vi "Fuse.vi"() -> ()   [LabVIEW 2010]
uses:
  PCAN/Labview/ControlCAN/ControlCAN.llb/CAN Channel.ctl
  PCAN/Labview/ControlCAN/ControlCAN.llb/DevType.ctl
  PCAN/Labview/ControlCAN/ControlCAN.llb/VCI_INIT_CONFIG.ctl
  PCAN/Labview/ControlCAN/ControlCAN.llb/InitFlag.ctl
  PCAN/Labview/ControlCAN/ControlCAN.llb/Fliter.ctl
  PCAN/Labview/ControlCAN/ControlCAN.llb/Mode.ctl
  PCAN/Labview/ControlCAN/ControlCAN.lvlib
panel:
  in  "Address":string="192.168.1.2"
  out "TX status":bool
  in  "stop Listen":bool
  in  "status":bool
  in  "Port":u16=8030
  out "conn ID":refnum<k5>
  in  "status 2":bool
  out "Config_CANAT":T7 {"DevType" items=["USB-CAN"=3, "USB-CAN2"=4]; "CanIndex" items=["通道1", "通道2"]; "VCI_INIT_CONFIG"."Fliter" items=["接收所有类型"=3, "只接收标准帧"=4, "只接收扩展帧"=7]; "VCI_INIT_CONFIG"."Mode" items=["正常工作", "自测模式（环回）", "仅侦听模式"]; "VCI_INIT_CONFIG"."InitFlag" items=["使用Flash参数", "使用界面设置参数"]}
  in  "Channel 2":T2 caption="Channel" items=["Channel 1", "Channel 2"]
  in  "CANType":u16(ring) items=["LAWICEL", "PCAN", "CANalystII", "TCP Client", "TCP Server"]
  in  "Get_Log_Time":i32=-1
  in  "Get_Log_Selector":bool
  out "Rcv_Msg":u8
  out "Send_Msg":bool
  in  "ParamFlagStop 2":bool
  out "error out 7":errorcluster
  in  "SysParamFlagStop":bool
  in  "System_Param_Time":i32=-1
  out "System Param Number":u8=9
  in  "System_Selector":bool
  in  "Ch_Selector":bool
  out "Param Nm":u8=9
  in  "ParamFlagStop":bool
  in  "Ch_Param_Time":i32=-1
  out "error out 2":errorcluster
  in  "Clear History":bool
  in  "Ring":u16(ring) items=["None", "Status", "ADC", "Status&ADC", "Temperature"]
  in  "Time":i32=-1
  out "History":string
  in  "Tab Control":T8(tab)
  in  "cleanPl":bool
  out "XY Graph":cluster{"Time":timestamp, "Data":dbl}[](graph)
  in  "Get Temp":bool
  out "Termistor":dbl format="%#.2g"
  in  "Control  Ch 1":bool
  in  "Status":bool
  in  "Trip Status":u16(ring) items=["Not tripped", "Tripped"]
  in  "Status":bool
  in  "Rsense":dbl
  in  "Gain":dbl
  in  "Get_ADC":bool
  out "ADC Units":dbl
  in  "Vin_Vout":bool
  out "Vin [V]":dbl
  out "Vout [V]":dbl
  in  "System Up Time  Set":u32
  in  "Unit Add Set":u32 format="%.0x"
  in  "R Sense [Ohms] Set":u32
  in  "Op Amp Gain Set":u32
  in  "Set System Params":bool
  in  "Retry Delay Set":u32
  in  "Number Of Retry Set":u32
  in  "Ch Received":u8
  in  "Set Channel Params":bool
  in  "Current Threshold [A] Set":u32
  in  "Channel On Delay [ms] Set":u32
  out "System Up Time":u32
  out "Unit Add":u32 format="%.0x"
  out "R Sense [Ohms]":u32
  out "Op Amp Gain":u32
  in  "Get System Params":bool
  out "Retry Delay":u32
  out "Number Of Retry":u32
  out "Ch Received":u8
  in  "Get Params":bool
  out "Current Threshold [A]":u32
  out "Channel On Delay [ms]":u32
  in  "Get Version":bool
  out "Unit PN":string
  out "SW ver":string
  in  "Clear Log":bool
  out "Event Logs":string
  in  "Get Log":bool
  in  "Clear Event Logs":bool
  out "Reset Fail":u32
  in  "Get Channel Protection":bool
  out "Channel Protection":string
  in  "Set Protection":u8(ring)=1 items=["No Protection"=3, "FF_OFF"=2, "ADC_OFF"=1, "All"=0]
  in  "Channel":u8(ring)=1 items=["Ch 1"=1, "Ch 2"=2, "Ch 3"=3, "Ch 4"=4, "Ch 5"=5, "Ch 6"=6, "Ch 7"=7, "Ch 8"=8]
  in  "Set Channel Protection":bool
  in  "TxID":u32 format="%x"
  in  "Data":u8[](array[numeric]) format="%.0x"
  in  "Sent Debug":bool
  out "MsgRX":T9 {"ID" format="%x"; "MSGTYPE" items=["STATUS"=128, "EXTENDED"=2, "RTR"=1, "DATA MSG"=0]; "aDATA" format="%x"}
  out "MsgTX":T9 {"ID" format="%x"; "MSGTYPE" items=["STATUS"=128, "EXTENDED"=2, "RTR"=1, "DATA MSG"=0]; "aDATA" format="%x"}
  in  "Channel":u8(ring)=1 items=["Ch 1"=1, "Ch 2"=2, "Ch 3"=3, "Ch 4"=4, "Ch 5"=5, "Ch 6"=6, "Ch 7"=7, "Ch 8"=8]
  in  "Get Reset count":bool
  out "Reset Counter":u32
  out "RX Cnt":u32
  out "TX Cnt":u32
  in  "stop m":bool
  out "error out 5":errorcluster
  out "error out 6":errorcluster
  out "erroro5 2":errorcluster
  out "erroro5":errorcluster
  out "error out 4":errorcluster
  out "VISA res_out":refnum<visa-resource-name>
  in  "Seria- Port":refnum<visa-resource-name>="COM5"
  out "error out 3":errorcluster
  out "error02":errorcluster
  out "error out":errorcluster
  out "RX":bool
  out "TX":bool
  in  "Disonnect":bool
  in  "Connect":bool
  out "CommIcon":bool=TRUE
  in  "UIFlagStop":bool
  in  "RXFlagStop":bool
  in  "IntFlagStop":bool
  in  "TXFlagStop":bool
  out "Error":string
  out "Adapter Version":string
  in  "type":i32(ring) items=["extended", "standart"]
  in  "baud":u16(ring)=20 items=["1M"=20, "500K"=28, "250K"=284, "125K"=796, "100K"=17199, "50K"=18223, "20K"=21295, "10K"=26415, "5K"=32639]
  # "[msec]"
  # "ver 0.0.1.b"
  # "Fuse Status"
  # "ADC"
  # "Temperature"
  # "Vin/Vout"
  # "Version"
  # "Channel Parameter"
  # "System Parameters"
  # "Channel Parameter"
  # "System Parameters"
  # "Custom Message"
  # "FF Reset Counter"
  # "Channel Protection"
  # "PowerRider CANBus interface"
  # "REDLER TECHNOLOGIES LTD"
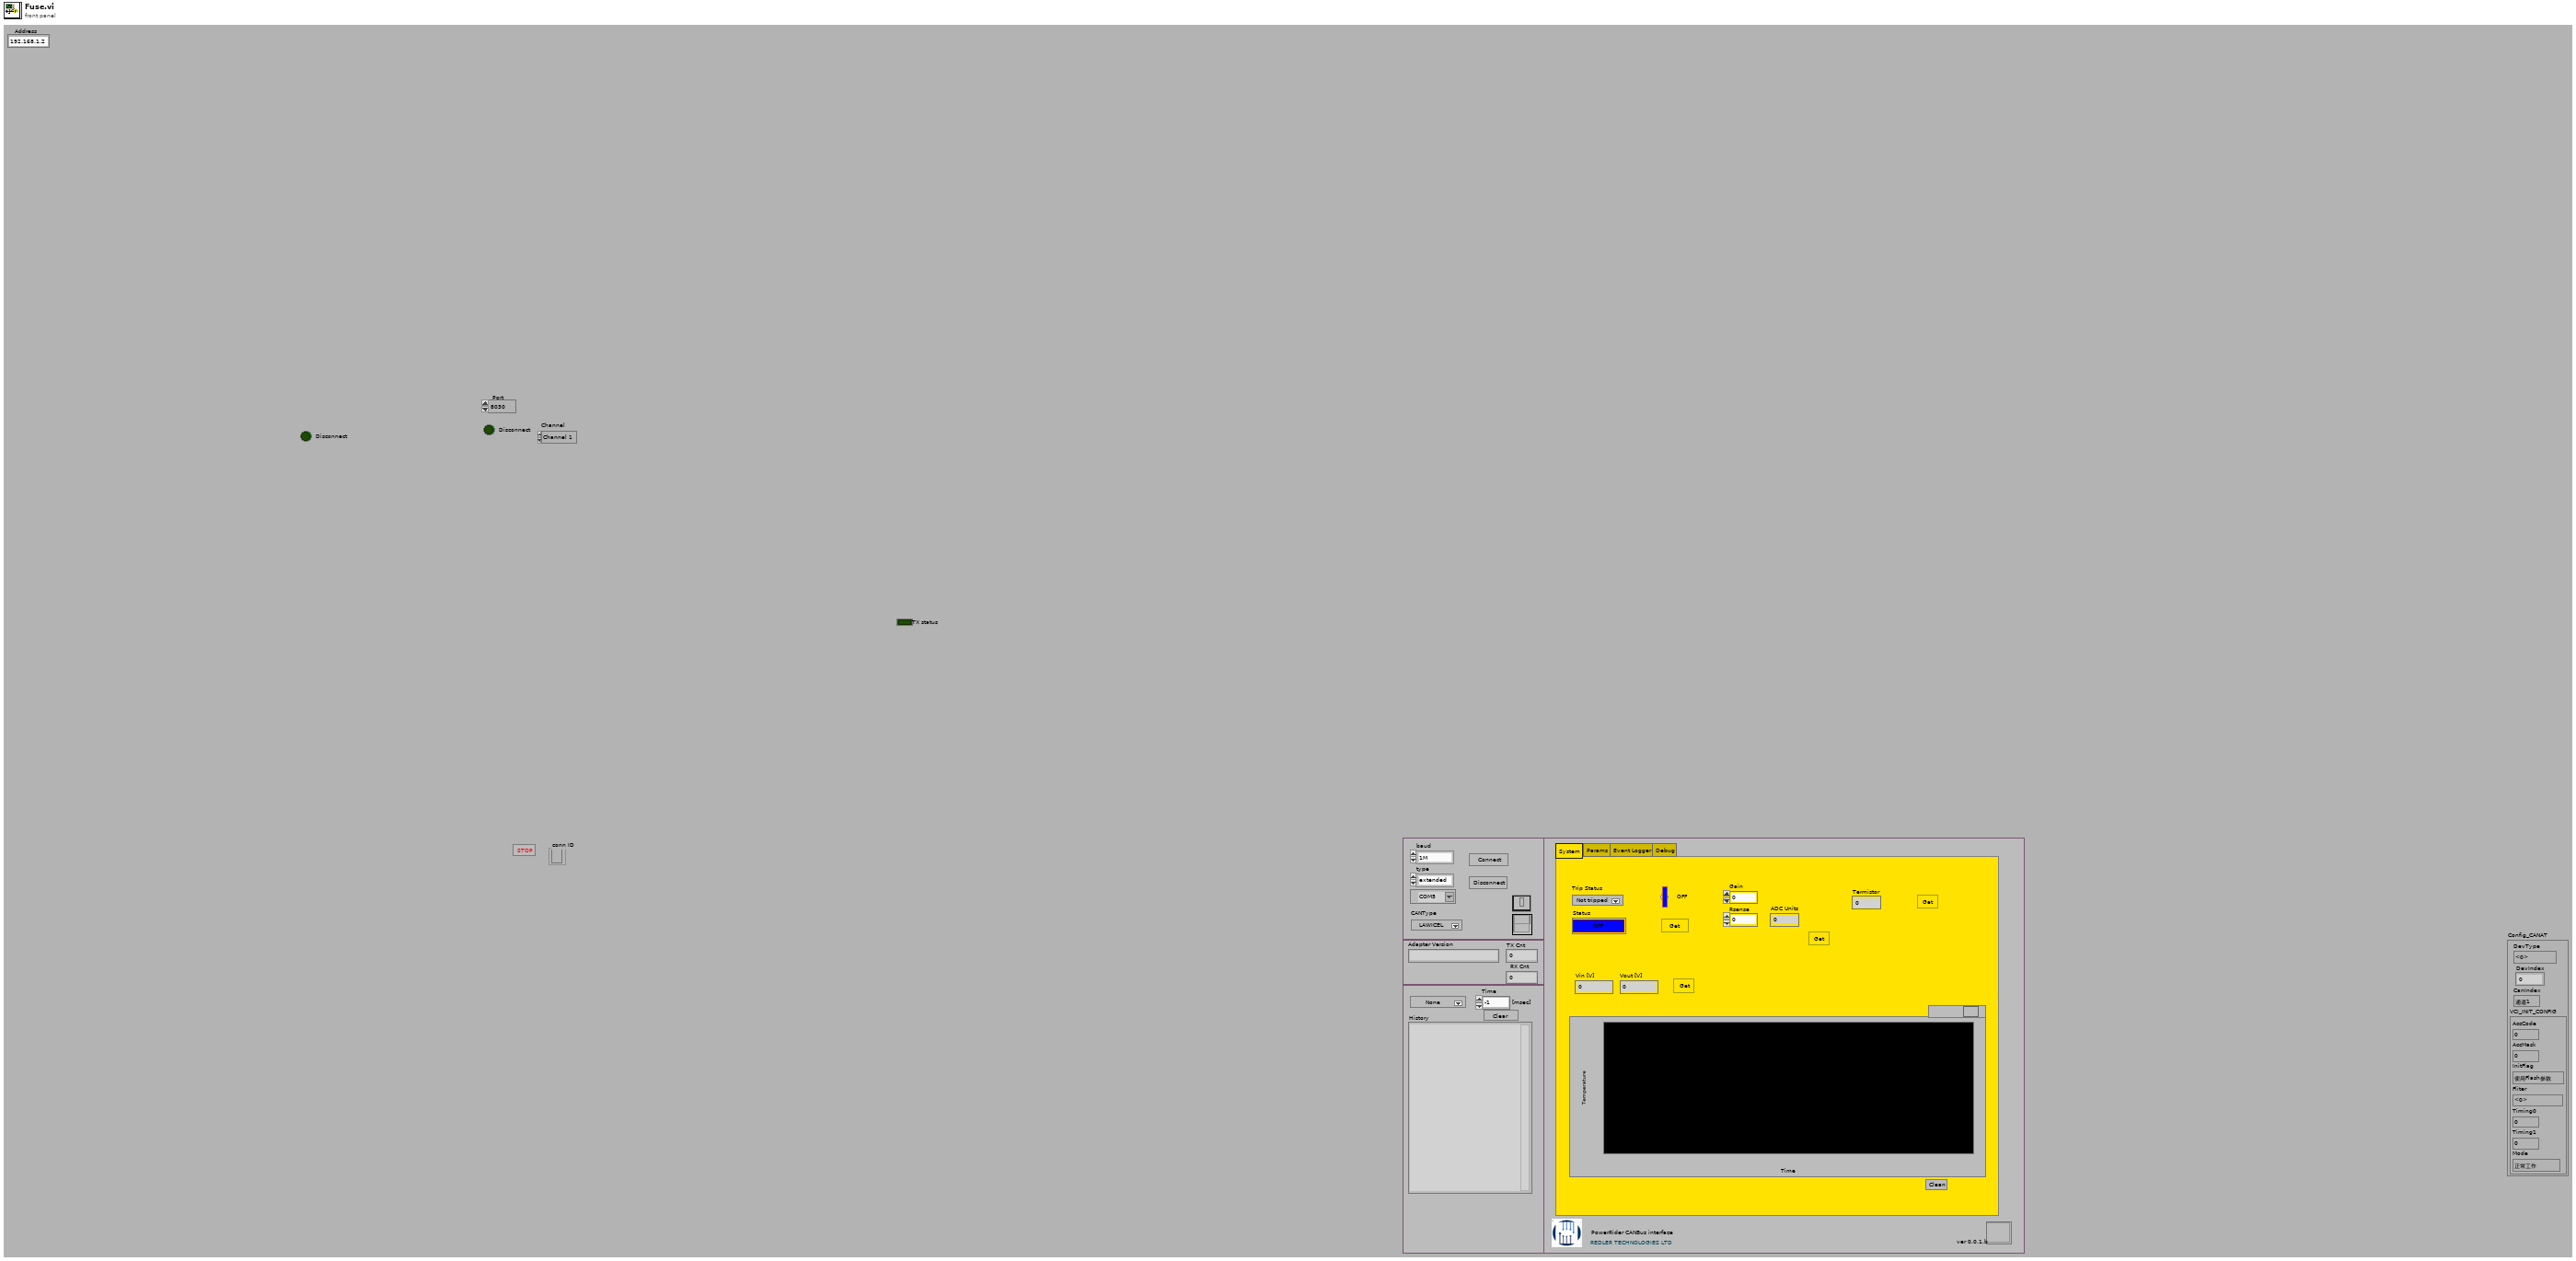
[diagram p1: front panel]
types:
  T1 = typedef "ControlCAN.lvlib/DevType.ctl" = u32
  T2 = typedef "ControlCAN.lvlib/CAN Channel.ctl" = u32
  T3 = typedef "ControlCAN.lvlib/VCI_INIT_CONFIG.ctl" = cluster{"AccCode":u32, "AccMask":u32, "InitFlag":T4, "Fliter":T5, "Timing0":u8, "Timing1":u8, "Mode":T6}
  T4 = typedef "ControlCAN.lvlib/InitFlag.ctl" = u32
  T5 = typedef "ControlCAN.lvlib/Fliter.ctl" = u8
  T6 = typedef "ControlCAN.lvlib/Mode.ctl" = u8
  T7 = cluster{"DevType":T1, "DevIndex":u32, "CanIndex":T2, "VCI_INIT_CONFIG":T3}
  T8 = enum32{"System", "Params", "Event Logger", "Debug"}
  T9 = cluster{"ID":u32, "MSGTYPE":u8, "LEN":u8, "aDATA":u8[]}
  T10 = typedef "PCAN_ERROR.ctl" = i32
  T11 = cluster{"Is Warning":bool, "Is Error":bool, "Message":string}
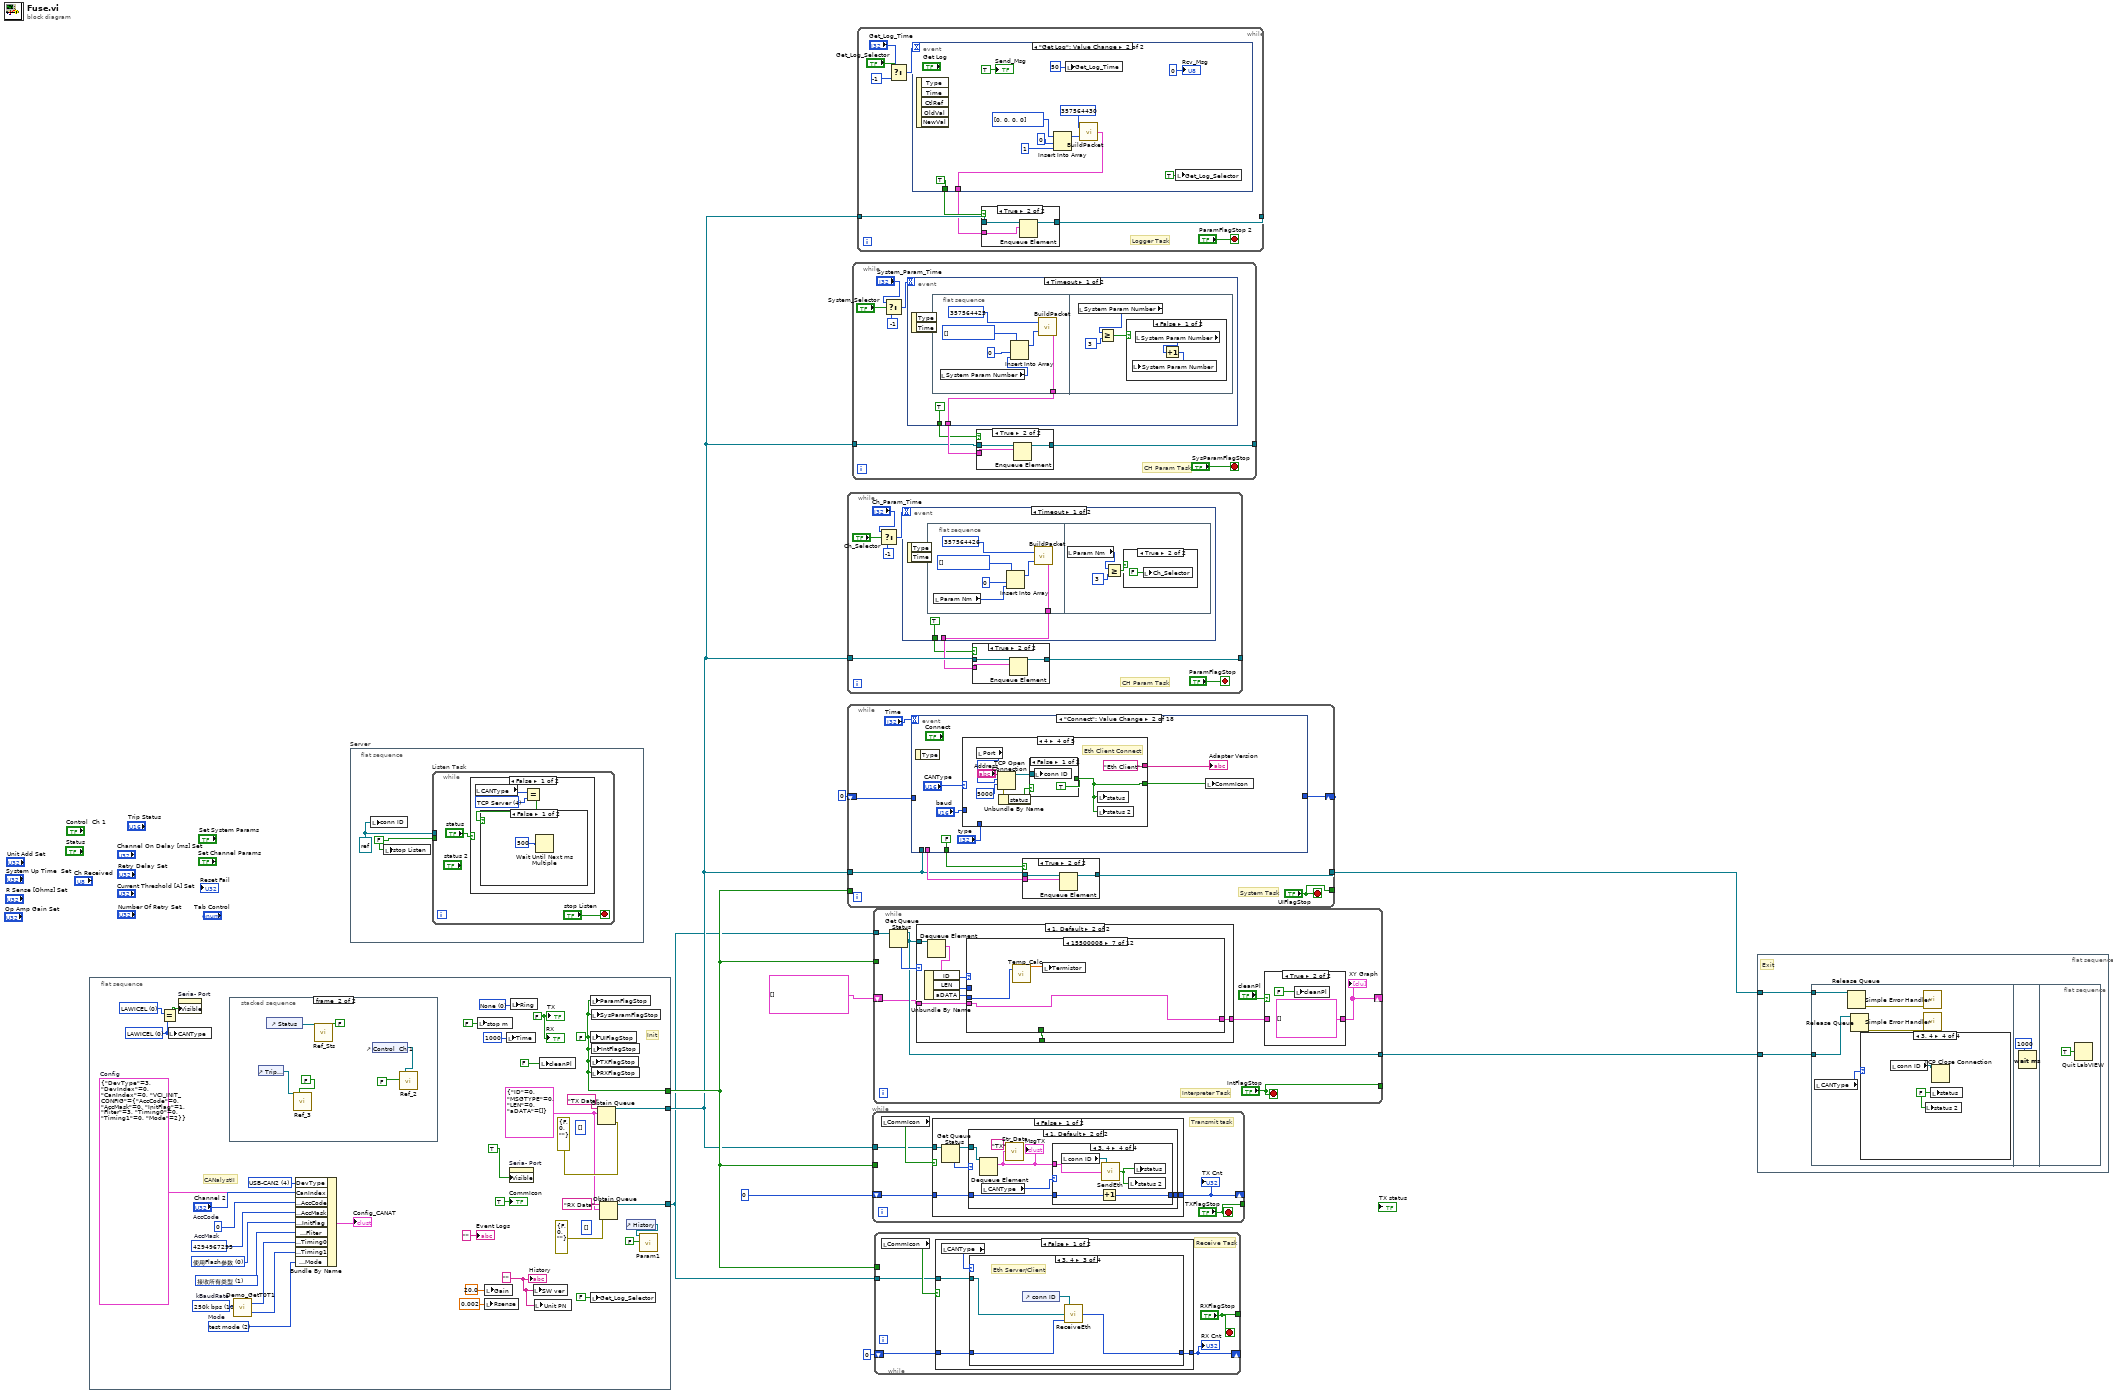
[diagram p0: block diagram]
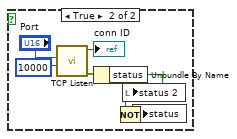
[diagram p2: hidden frame]
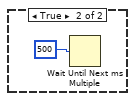
[diagram p3: hidden frame]
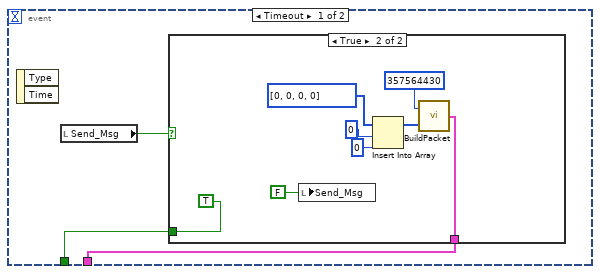
[diagram p4: hidden frame]
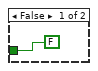
[diagram p5: hidden frame]
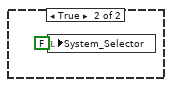
[diagram p7: hidden frame]
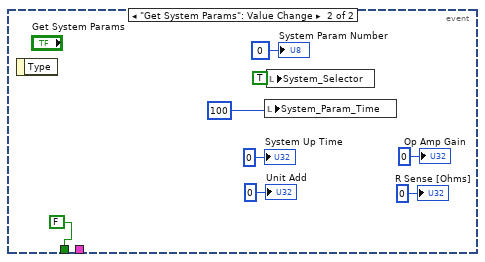
[diagram p8: hidden frame]
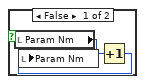
[diagram p10: hidden frame]
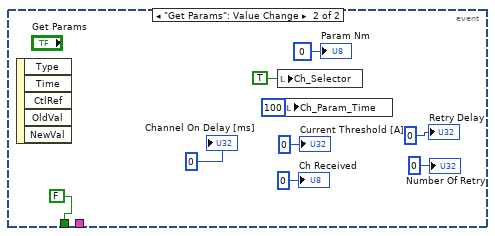
[diagram p11: hidden frame]
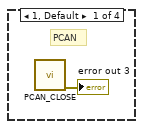
[diagram p13: hidden frame]
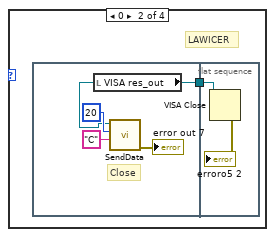
[diagram p14: hidden frame]
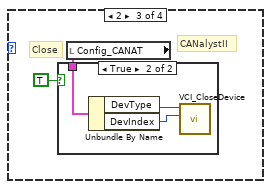
[diagram p15: hidden frame]
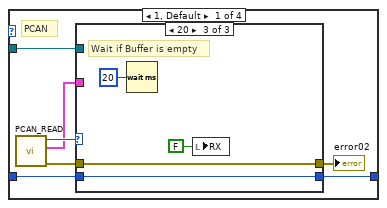
[diagram p17: hidden frame]
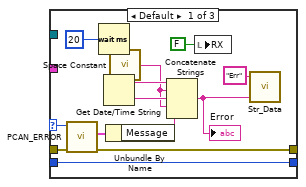
[diagram p18: hidden frame]
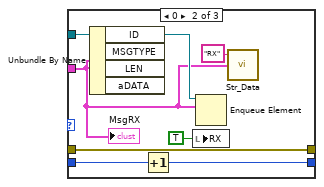
[diagram p19: hidden frame]
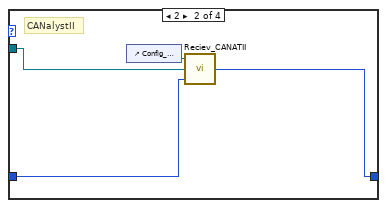
[diagram p20: hidden frame]
diagram:
  n1 = flat-sequence {
    tunnel: [w28] -> w9
    tunnel: [w42] -> w3
    tunnel: [w38] -> w1
    frame #0 {
      w11 = u16 0 items=["LAWICEL", "PCAN", "CANanlII"] ("CANType")
      w17 = u32 4294967295  # AccMask
      w18 = T4 0 items=["使用Flash参数", "使用界面设置参数"] ("InitFlag")
      w23 = T6 2 items=["normal operation", "Listen-only mode", "test mode"]  # Mode
      w19 = T5 1 items=["接收所有类型"=1, "只接收标准帧"=2, "只接收扩展帧"=3] ("Fliter")
      w20 = u8 10 items=["5k bps"=1, "10k bps"=2, "20k bps"=3, "40k bps"=4, "50k bps"=5, "80k bps"=6, "100k bps"=7, "125k bps"=8, "200k bps"=9, "250k bps"=10, "400k bps"=11, "500k bps"=12, "666k bps"=13, "800k bps"=14, "1000k bps"=15, "33.33k bps"=16, "66.66k bps"=17, "83.33k bps"=18]  # kBaudRate
      w16 = u32 0  # AccCode
      w14 = T1 4 items=["USB-CAN"=3, "USB-CAN2"=4] ("DevType")
      w13 = T7 {"DevType"=3, "DevIndex"=0, "CanIndex"=0, "VCI_INIT_CONFIG"={"AccCode"=0, "AccMask"=0, "InitFlag"=1, "Fliter"=3, "Timing0"=0, "Timing1"=0, "Mode"=2}}  # Config
      w12 = u16 0 items=["LAWICEL", "PCAN", "CANanlII"] ("CANType")
      w32 = u16 0 items=["None", "Status", "ADC", "Status&ADC"] ("Ring")
      w31 = "" ("str out")
      w39 = T9 {"ID"=0, "MSGTYPE"=0, "LEN"=0, "aDATA"=[]} ("Msg")
      w40 = FALSE ("TX")
      (unwired) u8[] []
      (unwired) u8[] []
      w28 = FALSE ("UIFlagStop")
      # "CANalystII"
      # "Init"
      n2 = Equal?(x=w11, y=w12) -> (x = y?=w10:bool)
      n3 = local write "CANType"(w12) -> ()
      n4 = property on="Seria- Port" class="VISAName"("Visible"=w10) -> ()  [unwired: 2 in, 2 out]
      n5 = stacked-sequence {
        frame #0 {
          n6 = local write "Control  Ch 1"(FALSE ("Control  Ch 1")) -> ()
          n7 = local write "Status"(FALSE ("Status")) -> ()
        }
        frame #1 {
          n8 = control-ref of="Trip Status"() -> (w50:refnum<vi>)
          n9 = control-ref of="Status"() -> (w52:refnum<vi>)
          n10 = call "Ref_3.vi"("Trip  Ch 1"=w50, "Init_F"=FALSE) -> ()  [unwired: 16 in, 10 out]
          n11 = call "Ref_Sts.vi"("Status Ch 1"=w52, "Init_F"=FALSE) -> ()  [unwired: 16 in, 10 out]
          n12 = control-ref of="Control  Ch 1"() -> (w54:refnum<vi>)
          n13 = call "Ref_2.vi"("Init_F"=FALSE, "Control  Ch 1"=w54) -> ()  [unwired: 15 in, 11 out]
        }
      }
      n14 = call "Demo_GetT0T1.vi"("kBaudRate"=w20) -> ("Timing0"=w21:u8, "Timing1"=w22:u8)
      n15 = Bundle By Name(cluster=w13, "DevType"=w14, "CanIndex"="Channel 2", "VCI_INIT_CONFIG.AccCode"=w16, "VCI_INIT_CONFIG.AccMask"=w17, "VCI_INIT_CONFIG.InitFlag"=w18, "VCI_INIT_CONFIG.Fliter"=w19, "VCI_INIT_CONFIG.Timing0"=w21, "VCI_INIT_CONFIG.Timing1"=w22, "VCI_INIT_CONFIG.Mode"=w23) -> (→"Config_CANAT":T7)
      n16 = local write "stop m"(FALSE ("stop m")) -> ()
      n17 = local write "Rsense"(0.002 ("Rsense")) -> ()
      n18 = local write "Gain"(20.0 ("Gain")) -> ()
      n19 = local write "Time"(1000 ("Time")) -> ()
      n20 = property on="Seria- Port" class="VISAName"("Visible"=TRUE ("CAN Type")) -> ()  [unwired: 2 in, 2 out]
      n21 = local write "Ring"(w32) -> ()
      n22 = local write "SW ver"(w31) -> ()
      n23 = local write "Unit PN"(w31) -> ()
      n24 = local write "cleanPl"(FALSE ("clean  Ch 2")) -> ()
      n25 = local write "ParamFlagStop"(w28) -> ()
      n26 = local write "UIFlagStop"(w28) -> ()
      n27 = local write "TXFlagStop"(w28) -> ()
      n28 = local write "Get_Log_Selector"(FALSE ("Get_Log_Selector")) -> ()
      n29 = local write "SysParamFlagStop"(w28) -> ()
      n30 = local write "RXFlagStop"(w28) -> ()
      n31 = local write "IntFlagStop"(w28) -> ()
      n32 = Obtain Queue(name (unnamed)="TX Data", element data type=w39, error in (no error)=errorcluster {"status"=FALSE, "code"=0, "source"=""}) -> (queue out=w42:refnum<queue>)  [unwired: 2 in, 2 out]
      n33 = Obtain Queue(name (unnamed)="RX Data", element data type=w39, error in (no error)=errorcluster {"status"=FALSE, "code"=0, "source"=""}) -> (queue out=w38:refnum<queue>)  [unwired: 2 in, 2 out]
      n34 = control-ref of="History"() -> (w34:refnum<vi>)
      n35 = call "Param1.vi"("str"=w34, "Init_F"=FALSE) -> ()  [unwired: 16 in, 2 out]
      "CommIcon" <- TRUE ("CommIcon")
      "RX" <- w40
      "TX" <- w40
      "History" <- w31
      "Event Logs" <- "" ("Event Logs")
    }
  }
  n36 = flat-sequence "Server" {
    frame #0 {
      w56 = refnum<k5> refnum ("connection ID")
      w55 = FALSE ("status")
      n37 = local write "conn ID"(w56) -> ()
      n38 = local write "stop Listen"(w55) -> ()
      n39 = while "Listen Task" {
        tunnel: w55 -> [_]
        tunnel: w56 -> [_]
        stop <- "stop Listen" stop-if-true
        n40 = case shown="False" "status" {
          frame False {
            w60 = u16 4 items=["LAWICEL", "PCAN", "CANalystII", "TCP Client", "TCP Server"] ("CANType 2")
            n41 = local read "CANType"() -> (w61:u16)
            n42 = Equal?(x=w61, y=w60) -> (x = y?=w59:bool)
            n43 = case shown="False" w59 {
              frame False {
                n44 = Wait Until Next ms Multiple(millisecond multiple=u32 500) -> ()  [unwired: 1 out]
              }
              frame True {
                n45 = call <vilib>:"TCP Listen.vi"("timeout ms (wait forever: -1)"=10000, "port"="Port") -> ("error out"=w66:errorcluster, "connection ID"=→"conn ID":refnum<k5>)  [unwired: 6 in, 2 out]
                n46 = Unbundle By Name(w66) -> ("status"=w63:bool)
                n47 = Not(x=w63) -> (.not. x?=w64:bool)
                n48 = local write "status 2"(w63) -> ()
                n49 = local write "status"(w64) -> ()
              }
            }
          }
          frame True {
            n50 = Wait Until Next ms Multiple(millisecond multiple=u32 500) -> ()  [unwired: 1 out]
          }
        }
      }
    }
  }
  n51 = while {
    tunnel: w3 -> [w77]
    tunnel: [w76] -> _
    stop <- "ParamFlagStop" stop-if-true
    # "CH Param Task"
    n52 = Select(t="Ch_Param_Time", s="Ch_Selector", f=-1) -> (s? t:f=w73:i32)
    n53 = event shown="[0] Timeout" {
      selector: _ -> [_ _]
      dyn-events: _ -> [_ _]
      timeout: w73 -> [_ _]
      tunnel: [w80 _] -> w72
      tunnel: [TRUE FALSE] -> w70
      event Timeout {
        n54 = event-data() -> ()  [unwired: 1 in, 2 out]
        n55 = flat-sequence {
          tunnel: [w86] -> w80
          frame #0 {
            n56 = local read "Param Nm"() -> (w81:u8)
            n57 = Insert Into Array(array=u8[] [] ("Data 2"), index=0, new element=w81) -> (w82:u8[])
            n58 = call "BuildPacket.vi"("Data"=w82, "TxID"=u32 357564426 ("Param ID")) -> ("MsgTX 2"=w86:T9)
          }
          frame #1 {
            n59 = local read "Param Nm"() -> (w89:u8)
            n60 = Greater Or Equal?(x=w89, y=u8 3) -> (x >= y?=w88:bool)
            n61 = case shown="True" w88 {
              frame False {
                n62 = local read "Param Nm"() -> (w91:u8)
                n63 = Increment(x=w91) -> (x+1=w90:u8)
                n64 = local write "Param Nm"(w90) -> ()
              }
              frame True {
                n65 = local write "Ch_Selector"(FALSE ("Timer Select")) -> ()
              }
            }
          }
        }
      }
      event "Get Params": Value Change {
        n66 = event-data() -> ()  [unwired: 1 in, 5 out]
        n67 = local write "Ch_Selector"(TRUE ("Timer Select")) -> ()
        n68 = local write "Ch_Param_Time"(100 ("Time Param")) -> ()
        "Param Nm" <- u32 0 ("Param ID")
        "Current Threshold [A]" <- u32 0 ("Current Threshold [A]")
        "Ch Received" <- u8 0 ("Ch Received")
        "Channel On Delay [ms]" <- u32 0 ("Channel On Delay [ms]")
        "Number Of Retry" <- u32 0 ("Ch Received")
        "Retry Delay" <- u32 0 ("Current Threshold [A]")
      }
    }
    n69 = case shown="True" w70 {
      tunnel: w77 -> [w102 w105]
      tunnel: [w102 w104] -> w76
      tunnel: w72 -> [_ w103]
      frame False {
      }
      frame True {
        n70 = Enqueue Element(queue=w105, element=w103) -> (queue out=w104:refnum<queue>)  [unwired: 1 in, 3 out]
      }
    }
  }
  n71 = while {
    tunnel: w9 -> [_]
    tunnel: ["UIFlagStop"] -> _
    tunnel: w3 -> [w107]
    tunnel: [w106] -> w8
    shift-right: [w108] -> _
    shift-left: u32 0 -> [w109]
    stop <- "UIFlagStop" stop-if-true
    # "System Task"
    n72 = event shown="[1] \"Connect\": Value Change" {
      selector: _ -> [_ _ _ _ _ _ _ _ _ _ _ _ _ _ _ _ _ _]
      dyn-events: _ -> [_ _ _ _ _ _ _ _ _ _ _ _ _ _ _ _ _ _]
      timeout: "Time" -> [_ _ _ _ _ _ _ _ _ _ _ _ _ _ _ _ _ _]
      tunnel: [w121 _ _ w192 w197 _ w205 w211 w218 w222 w228 w245 w255 w259 _ _ _ w287] -> w112
      tunnel: [w122 FALSE FALSE TRUE TRUE FALSE TRUE TRUE TRUE TRUE TRUE TRUE TRUE TRUE FALSE FALSE _ TRUE] -> w111
      tunnel: w109 -> [w119 _ _ _ _ w202 _ _ _ _ _ _ _ _ _ _ _ _]
      tunnel: [w118 _ _ _ _ w202 _ _ _ _ _ _ _ _ _ _ _ _] -> w108
      tunnel: w107 -> [_ _ _ _ _ _ _ _ _ _ _ _ _ _ _ _ _ _]
      event Timeout {
        n73 = event-data() -> ()  [unwired: 1 in, 1 out]
        n74 = case shown="3" "Ring" {
          tunnel: [FALSE TRUE TRUE TRUE] -> w122
          tunnel: [T9 {"ID"=0, "MSGTYPE"=0, "LEN"=0, "aDATA"=[]} ("Msg") w127 w132 w138] -> w121
          tunnel: w119 -> [_ _ _ w140]
          tunnel: [u32 0 u32 0 u32 0 w136] -> w118
          frame 0, Default {
          }
          frame 1 {
            w129 = u32 357564416  # ID
            # "Status"
            n75 = call "BuildPacket.vi"("Data"=u8[] [] ("Data 2"), "TxID"=w129) -> ("MsgTX 2"=w127:T9)
          }
          frame 2 {
            w133 = u32 357564419  # ID
            # "ADC"
            n76 = call "BuildPacket.vi"("Data"=u8[] [] ("Data 2"), "TxID"=w133) -> ("MsgTX 2"=w132:T9)
          }
          frame 3 {
            n77 = case shown="1" w140 {
              selector: w140 -> [w143 _]
              tunnel: [w144 w146] -> w137
              tunnel: [w142 u32 0] -> w136
              frame 0, Default {
                w144 = u32 357826560  # ID
                # "Status"
                n78 = Increment(x=w143) -> (x+1=w142:u32)
              }
              frame 1 {
                w146 = u32 357564419  # ID
                # "ADC"
              }
            }
            n79 = call "BuildPacket.vi"("Data"=u8[] [] ("Data 2"), "TxID"=w137) -> ("MsgTX 2"=w138:T9)
          }
        }
      }
      event "Connect": Value Change {
        n80 = event-data() -> ()  [unwired: 1 in, 1 out]
        n81 = case shown="4" "CANType" {
          tunnel: [w155 w162 w168 w171 w182] -> w151
          tunnel: [w157 "CANalystII" ("read ver") "" ("read ver") "Eth Client" ("read ver") w183] -> w150
          tunnel: "baud" -> [w154 w161 _ _ w181]
          tunnel: "type" -> [w153 w160 _ _ _]
          frame 1, Default {
            # "PCAN"
            n82 = call "Init_PCAN.vi"("type"=w153, "baud"=w154) -> ("Boolean"=w156:bool, "Version"=w157:string)
            n83 = Not(x=w156) -> (.not. x?=w155:bool)
          }
          frame 2 {
            # "CANalystII"
            n84 = flat-sequence {
              tunnel: w161 -> [w165]
              tunnel: w160 -> [_]
              tunnel: [w164] -> w158
              tunnel: [w167] -> w159
              tunnel: w158 -> [w166]
              frame #0 {
                n85 = control-ref of="Config_CANAT"() -> (w164:refnum<vi>)
                n86 = call "ChangeCANBaud.vi"("baud in"=w165, "reference"=w164) -> ()
              }
              frame #1 {
                n87 = call "InitCAN_ATII.vi"("Config"=w166) -> ("Sts"=w167:bool)
              }
            }
            n88 = Not(x=w159) -> (.not. x?=w162:bool)
          }
          frame 3 {
            # "Eth Server Connect"
            n89 = local read "CommIcon"() -> (w168:bool)
          }
          frame 4 {
            # "Eth Client Connect"
            n90 = local read "Port"() -> (w175:u16)
            n91 = TCP Open Connection(address="Address", remote port or service name=w175, timeout ms (60000)=5000) -> (connection ID=w177:refnum<k5>, error out=w173:errorcluster)  [unwired: 1 in, 1 out]
            n92 = Unbundle By Name(w173) -> ("status"=w176:bool)
            n93 = case shown="False" w176 {
              tunnel: w177 -> [w179 _]
              tunnel: [TRUE FALSE] -> w171
              frame False {
                n94 = local write "conn ID"(w179) -> ()
              }
              frame True {
              }
            }
            n95 = local write "status"(w171) -> ()
            n96 = local write "status 2"(w171) -> ()
          }
          frame 0 {
            # "LAWICER"
            n97 = call "Init_Lawicel.vi"("baud"=w181, "Seria- Port"="Seria- Port") -> ("error out 4"=→"error out 4":errorcluster, "Status"=w184:bool, "read ver"=w183:string, "VISA res_out"=→"VISA res_out":refnum<visa-resource-name>)  [unwired: 1 in]
            n98 = Not(x=w184) -> (.not. x?=w182:bool)
          }
        }
        "Adapter Version" <- w150
        n99 = local write "CommIcon"(w151) -> ()
      }
      event "stop m": Value Change {
        w188 = TRUE ("UIFlagStop")
        n100 = event-data() -> ()  [unwired: 1 in, 1 out]
        n101 = local write "UIFlagStop"(w188) -> ()
        n102 = local write "TXFlagStop"(w188) -> ()
        n103 = local write "RXFlagStop"(w188) -> ()
        n104 = local write "IntFlagStop"(w188) -> ()
        n105 = local write "SysParamFlagStop"(w188) -> ()
        n106 = local write "ParamFlagStop"(w188) -> ()
      }
      event "Sent Debug": Value Change {
        n107 = event-data() -> ()  [unwired: 1 in, 1 out]
        n108 = call "BuildPacket.vi"("Data"="Data", "TxID"="TxID") -> ("MsgTX 2"=w192:T9)
      }
      event "Get Version": Value Change {
        w194 = "" ("SW ver")
        w195 = u32 357564423  # ID
        # "0x15500007"
        n109 = event-data() -> ()  [unwired: 1 in, 1 out]
        n110 = call "BuildPacket.vi"("Data"=u8[] [] ("Data 2"), "TxID"=w195) -> ("MsgTX 2"=w197:T9)
        "SW ver" <- w194
        "Unit PN" <- w194
      }
      event "CANType": Value Change {
        w200 = u16 0 items=["LAWICEL", "PCAN", "CANanlII"] ("CANType")
        n111 = event-data() -> ()  [unwired: 1 in, 1 out]
        n112 = local read "CANType"() -> (w201:u16)
        n113 = Equal?(x=w200, y=w201) -> (x = y?=w199:bool)
        n114 = property on="Seria- Port" class="VISAName"("Visible"=w199) -> ()  [unwired: 2 in, 2 out]
      }
      event "Get Temp": Value Change {
        w206 = u32 357564424  # ID
        # "0x15500008"
        n115 = event-data() -> ()  [unwired: 1 in, 1 out]
        n116 = call "BuildPacket.vi"("Data"=u8[] [] ("Data 2"), "TxID"=w206) -> ("MsgTX 2"=w205:T9)
        "Termistor" <- 0.0 ("CPU Temp")
      }
      event "Status": Value Change {
        w209 = u32 357564416  # ID
        # "Status"
        # "0x1550000"
        n117 = event-data() -> ()  [unwired: 1 in, 1 out]
        n118 = call "BuildPacket.vi"("Data"=u8[] [] ("Data 2"), "TxID"=w209) -> ("MsgTX 2"=w211:T9)
      }
      event "Vin_Vout": Value Change {
        w217 = u32 357564420  # ID
        # "0x15500004"
        n119 = event-data() -> ()  [unwired: 1 in, 1 out]
        n120 = Insert Into Array(array=u8[] [] ("Data 2"), index=0, new element=u8 0 ("new element/subarray")) -> (w214:u8[])
        n121 = call "BuildPacket.vi"("Data"=w214, "TxID"=w217) -> ("MsgTX 2"=w218:T9)
      }
      event "Get Reset count": Value Change {
        w226 = u32 357564427  # ID
        # "0x1550000B"
        n122 = event-data() -> ()  [unwired: 1 in, 1 out]
        n123 = Insert Into Array(array=u8[] [] ("Data 2"), index=0, new element="Channel") -> (w224:u8[])
        n124 = call "BuildPacket.vi"("Data"=w224, "TxID"=w226) -> ("MsgTX 2"=w222:T9)
      }
      event "Set Channel Protection": Value Change {
        w238 = u32 357564428  # ID
        n125 = event-data() -> ()  [unwired: 1 in, 1 out]
        n126 = String To Byte Array(string="S") -> (unsigned byte array=w231:u8[])
        n127 = Index Array(array=w231, index=0) -> (element=w229:u8)
        n128 = Insert Into Array(array=u8[] [] ("Data 2"), index=0, new element #1="Channel", new element #2="Set Protection", new element #3=w229) -> (w236:u8[])
        n129 = call "BuildPacket.vi"("Data"=w236, "TxID"=w238) -> ("MsgTX 2"=w228:T9)
      }
      event "Get Channel Protection": Value Change {
        w246 = u32 357564428  # ID
        n130 = event-data() -> ()  [unwired: 1 in, 1 out]
        n131 = local read "Set Protection"() -> (w240:u8)
        n132 = local read "Channel"() -> (w241:u8)
        n133 = Insert Into Array(array=u8[] [] ("Data 2"), index=0, new element #1=w241, new element #2=w240, new element #3=u8 0 ("new element/subarray")) -> (w247:u8[])
        n134 = call "BuildPacket.vi"("Data"=w247, "TxID"=w246) -> ("MsgTX 2"=w245:T9)
        n135 = local write "Channel Protection"("" ("Channel Protection")) -> ()
      }
      event "Get_ADC": Value Change {
        w254 = u32 357564418  # ID
        # "ADC"
        n136 = event-data() -> ()  [unwired: 1 in, 5 out]
        n137 = Insert Into Array(array=u8[] [] ("Data 2"), index=0, new element=u8 0 ("new element/subarray")) -> (w251:u8[])
        n138 = call "BuildPacket.vi"("Data"=w251, "TxID"=w254) -> ("MsgTX 2"=w255:T9)
        "ADC Units" <- 0.0 ("ADC Value")
      }
      event "Control  Ch 1": Value Change {
        w258 = u32 357564417  # ID
        # "Channel control"
        # "0xAAA00001"
        n139 = event-data() -> ()  [unwired: 1 in, 1 out]
        n140 = call "CmdControl.vi"() -> ("Dataout"=w257:u8[])  [unwired: 4 in]
        n141 = call "BuildPacket.vi"("Data"=w257, "TxID"=w258) -> ("MsgTX 2"=w259:T9)
      }
      event "Disonnect": Value Change {
        n142 = event-data() -> ()  [unwired: 1 in, 1 out]
        n143 = local read "CANType"() -> (w261:u16)
        n144 = case shown="3, 4" w261 {
          tunnel: [TRUE TRUE TRUE TRUE] -> w262
          frame 1, Default {
            # "PCAN"
            n145 = call "PCAN_CLOSE.vi"() -> ()  [unwired: 1 in, 11 out]
          }
          frame 2 {
            # "CANalystII"
            # "Close"
            n146 = local read "Config_CANAT"() -> (w266:T7)
            n147 = case shown="True" TRUE {
              tunnel: w266 -> [_ w268]
              frame False {
              }
              frame True {
                n148 = Unbundle By Name(w268) -> ("DevType"=w270:T1, "DevIndex"=w269:u32)
                n149 = call "VCI_CloseDevice.vi"("DevIndex"=w269, "DevType"=w270) -> ()  [unwired: 1 in, 9 out]
              }
            }
          }
          frame 3, 4 {
            w271 = FALSE ("status")
            n150 = local read "conn ID"() -> (w272:refnum<k5>)
            n151 = local write "status 2"(w271) -> ()
            n152 = local write "status"(w271) -> ()
            n153 = TCP Close Connection(connection ID=w272) -> ()  [unwired: 2 in, 2 out]
          }
          frame 0 {
            # "LAWICER"
            n154 = flat-sequence {
              tunnel: [w277] -> w274
              tunnel: w274 -> [w281]
              frame #0 {
                # "Close"
                n155 = local read "VISA res_out"() -> (w277:refnum<visa-resource-name>)
                n156 = call "SendData.vi"("String"="C", "byte count"=u32 20, "VISA resource name out 2"=w277) -> ("error out"=→"error out 2":errorcluster)  [unwired: 1 in, 3 out]
              }
              frame #1 {
                n157 = VISA Close(VISA resource name=w281) -> (error out=→"erroro5":errorcluster)  [unwired: 1 in]
              }
            }
          }
        }
        n158 = local write "CommIcon"(w262) -> ()
      }
      event "Clear History": Value Change {
        n159 = event-data() -> ()  [unwired: 1 in, 1 out]
        n160 = local write "History"("" ("str out")) -> ()
      }
      event "Clear Event Logs": Value Change {
        n161 = event-data() -> ()  [unwired: 1 in, 5 out]
        n162 = local write "Event Logs"("" ("Event Logs")) -> ()
      }
      event "Clear Log": Value Change {
        n163 = event-data() -> ()  [unwired: 1 in, 5 out]
        n164 = flat-sequence {
          tunnel: [w288] -> w285
          tunnel: [w293] -> w287
          tunnel: w285 -> [w292]
          frame #0 {
            n165 = Two Button Dialog(message="Are you sure you want to erase the event logger", 1:"Cancel" ("F button name (\"Cancel\")"), 2:"OK" ("T button name (\"OK\")")) -> (T button?=w288:bool)
          }
          frame #1 {
            n166 = case shown="False" w292 {
              tunnel: [_ w297] -> w293
              frame False {
              }
              frame True {
                w301 = u32 357564430  # ID
                n167 = local write "Rcv_Msg"(u8 3 ("Rcv_Msg")) -> ()
                n168 = Insert Into Array(array=u8[] [] ("Data 2"), index=0, new element=u8 2 ("new element/subarray")) -> (w298:u8[])
                n169 = local write "Event Logs"("Erasing EEPROM please wait..." ("Event Logs")) -> ()
                n170 = call "BuildPacket.vi"("Data"=w298, "TxID"=w301) -> ("MsgTX 2"=w297:T9)
              }
            }
          }
        }
      }
    }
    n171 = case shown="True" w111 {
      tunnel: w107 -> [w114 w117]
      tunnel: [w114 w116] -> w106
      tunnel: w112 -> [_ w115]
      frame False {
      }
      frame True {
        n172 = Enqueue Element(queue=w117, element=w115) -> (queue out=w116:refnum<queue>)  [unwired: 1 in, 3 out]
      }
    }
  }
  n173 = while {
    tunnel: [w309] -> _
    tunnel: w3 -> [w302]
    stop <- "SysParamFlagStop" stop-if-true
    # "CH Param Task"
    n174 = Select(t="System_Param_Time", s="System_Selector", f=-1) -> (s? t:f=w306:i32)
    n175 = event shown="[0] Timeout" {
      selector: _ -> [_ _]
      dyn-events: _ -> [_ _]
      timeout: w306 -> [_ _]
      tunnel: [w312 _] -> w305
      tunnel: [TRUE FALSE] -> w303
      event Timeout {
        n176 = event-data() -> ()  [unwired: 1 in, 2 out]
        n177 = flat-sequence {
          tunnel: [w318] -> w312
          frame #0 {
            n178 = local read "System Param Number"() -> (w313:u8)
            n179 = Insert Into Array(array=u8[] [] ("Data 2"), index=0, new element=w313) -> (w314:u8[])
            n180 = call "BuildPacket.vi"("Data"=w314, "TxID"=u32 357564425 ("Param ID")) -> ("MsgTX 2"=w318:T9)
          }
          frame #1 {
            n181 = local read "System Param Number"() -> (w319:u8)
            n182 = Greater Or Equal?(x=w319, y=u8 3) -> (x >= y?=w321:bool)
            n183 = case shown="False" w321 {
              frame False {
                n184 = local read "System Param Number"() -> (w323:u8)
                n185 = Increment(x=w323) -> (x+1=w322:u8)
                n186 = local write "System Param Number"(w322) -> ()
              }
              frame True {
                n187 = local write "System_Selector"(FALSE ("Timer Select")) -> ()
              }
            }
          }
        }
      }
      event "Get System Params": Value Change {
        n188 = event-data() -> ()  [unwired: 1 in, 1 out]
        n189 = local write "System_Param_Time"(100 ("Time Param")) -> ()
        n190 = local write "System_Selector"(TRUE ("Timer Select")) -> ()
        "System Param Number" <- u8 0 ("Param ID")
        "System Up Time" <- u32 0 ("System Up Time  Out")
        "Unit Add" <- u32 0 ("Unit Add Out")
        "R Sense [Ohms]" <- u32 0 ("R Sense [Ohms] out")
        "Op Amp Gain" <- u32 0 ("Op Amp Gain out")
      }
    }
    n191 = case shown="True" w303 {
      tunnel: w302 -> [w333 w334]
      tunnel: [w333 w336] -> w309
      tunnel: w305 -> [_ w335]
      frame False {
      }
      frame True {
        n192 = Enqueue Element(queue=w334, element=w335) -> (queue out=w336:refnum<queue>)  [unwired: 1 in, 3 out]
      }
    }
  }
  n193 = while {
    tunnel: w3 -> [w344]
    tunnel: [w343] -> _
    stop <- "ParamFlagStop 2" stop-if-true
    # "Logger Task"
    n194 = Select(t="Get_Log_Time", s="Get_Log_Selector", f=-1) -> (s? t:f=w340:i32)
    n195 = event shown="[1] \"Get Log\": Value Change" {
      selector: _ -> [_ _]
      dyn-events: _ -> [_ _]
      timeout: w340 -> [_ _]
      tunnel: [w346 TRUE] -> w339
      tunnel: [w347 w359] -> w337
      event Timeout {
        n196 = event-data() -> ()  [unwired: 1 in, 2 out]
        n197 = local read "Send_Msg"() -> (w348:bool)
        n198 = case shown="True" w348 {
          tunnel: [_ w353] -> w347
          tunnel: [FALSE TRUE] -> w346
          frame False {
          }
          frame True {
            n199 = local write "Send_Msg"(FALSE ("End_Of_Log")) -> ()
            n200 = Insert Into Array(array=u8[] [0, 0, 0, 0] ("Data 2"), index=0, new element=u8 0 ("new element/subarray")) -> (w354:u8[])
            n201 = call "BuildPacket.vi"("Data"=w354, "TxID"=u32 357564430 ("Param ID")) -> ("MsgTX 2"=w353:T9)
          }
        }
      }
      event "Get Log": Value Change {
        n202 = event-data() -> ()  [unwired: 1 in, 5 out]
        n203 = Insert Into Array(array=u8[] [0, 0, 0, 0] ("Data 2"), index=0, new element=u8 1 ("new element/subarray")) -> (w360:u8[])
        n204 = local write "Get_Log_Time"(50 ("Time Param 3")) -> ()
        n205 = call "BuildPacket.vi"("Data"=w360, "TxID"=u32 357564430 ("Param ID")) -> ("MsgTX 2"=w359:T9)
        n206 = local write "Get_Log_Selector"(TRUE ("Get_Log_Timer")) -> ()
        "Rcv_Msg" <- u8 0 ("Rcv_Msg")
        "Send_Msg" <- TRUE ("Get_Log_Timer")
      }
    }
    n207 = case shown="True" w339 {
      tunnel: w344 -> [w369 w372]
      tunnel: [w369 w371] -> w343
      tunnel: w337 -> [_ w370]
      frame False {
      }
      frame True {
        n208 = Enqueue Element(queue=w372, element=w370) -> (queue out=w371:refnum<queue>)  [unwired: 1 in, 3 out]
      }
    }
  }
  n209 = while {
    tunnel: w9 -> [_]
    tunnel: ["TXFlagStop"] -> _
    tunnel: w3 -> [w375]
    shift-right: [w373] -> _
    shift-left: u32 0 -> [w374]
    stop <- "TXFlagStop" stop-if-true
    # "Transmit task"
    n210 = local read "CommIcon"() -> (w376:bool)
    n211 = case shown="False" w376 {
      tunnel: w375 -> [w382 _]
      tunnel: w374 -> [w379 w412]
      tunnel: [w378 w412] -> w373
      frame False {
        n212 = Get Queue Status(queue=w382) -> (queue out=w380:refnum<queue>, # elements in queue=w381:i32)  [unwired: 1 in, 7 out]
        n213 = case shown="1, Default" w381 {
          tunnel: w380 -> [_ w391]
          tunnel: w379 -> [w383 w390]
          tunnel: [w383 w389] -> w378
          frame 0 {
            n214 = local write "TX"(FALSE ("TX")) -> ()
            n215 = Wait (ms)(milliseconds to wait=u32 10) -> ()  [unwired: 1 out]
          }
          frame 1, Default {
            n216 = Dequeue Element(queue=w391) -> (element=w387:T9)  [unwired: 1 in, 4 out]
            "MsgTX" <- w387
            n217 = local read "CANType"() -> (w386:u16)
            n218 = call "Str_Data.vi"("Msg"=w387, "string"="TX") -> ()  [unwired: 1 in, 1 out]
            n219 = case shown="3, 4" w386 {
              tunnel: w387 -> [w396 w401 w403 w409]
              tunnel: w390 -> [w393 w398 w406 w411]
              tunnel: [w392 w397 w405 w410] -> w389
              frame 1, Default {
                # "PCAN"
                n220 = Increment(x=w393) -> (x+1=w392:u32)
                n221 = call "PCAN_WRITE.vi"("TPCANMsg"=w396) -> ("error out"=→"error out":errorcluster)  [unwired: 2 in, 8 out]
                n222 = local write "TX"(TRUE ("TX")) -> ()
              }
              frame 0 {
                # "LAWICER"
                n223 = Increment(x=w398) -> (x+1=w397:u32)
                n224 = local read "VISA res_out"() -> (w400:refnum<visa-resource-name>)
                n225 = call "SendData_CANUSB.vi"("Msg"=w401, "VISA res_in"=w400) -> ("error out 6"=→"error out 6":errorcluster)  [unwired: 1 in, 2 out]
                n226 = local write "TX"(TRUE ("TX")) -> ()
              }
              frame 2 {
                # "CANalystII"
                n227 = control-ref of="Config_CANAT"() -> (w404:refnum<vi>)
                n228 = Increment(x=w406) -> (x+1=w405:u32)
                n229 = call "Send_CAN_ATII.vi"("MsgTX"=w403, "Config"=w404) -> ()
              }
              frame 3, 4 {
                n230 = local read "conn ID"() -> (w408:refnum<k5>)
                n231 = Increment(x=w411) -> (x+1=w410:u32)
                n232 = call "SendEth.vi"("Msg"=w409, "conn ID"=w408) -> ("status"=w407:bool)  [unwired: 3 in]
                n233 = local write "status 2"(w407) -> ()
                n234 = local write "status"(w407) -> ()
              }
            }
          }
        }
      }
      frame True {
        n235 = Wait (ms)(milliseconds to wait=u32 10) -> ()  [unwired: 1 out]
      }
    }
    "TX Cnt" <- w373
  }
  n236 = while {
    tunnel: w9 -> [_]
    tunnel: ["IntFlagStop"] -> _
    tunnel: w1 -> [w421]
    tunnel: [w418] -> w7
    shift-right: [w414] -> _
    shift-left: cluster{"Time":timestamp, "Data":dbl}[] [] -> [w417]
    stop <- "IntFlagStop" stop-if-true
    # "Interpreter Task"
    n237 = Get Queue Status(queue=w421) -> (queue out=w418:refnum<queue>, # elements in queue=w420:i32)  [unwired: 1 in, 7 out]
    n238 = case shown="1, Default" w420 {
      tunnel: w418 -> [_ w434]
      tunnel: [_ w429] -> _
      tunnel: w417 -> [w425 w428]
      tunnel: [w425 w427] -> w415
      frame 0 {
        n239 = Wait (ms)(milliseconds to wait=u32 10) -> ()  [unwired: 1 out]
      }
      frame 1, Default {
        n240 = Dequeue Element(queue=w434) -> (element=w433:T9)  [unwired: 1 in, 4 out]
        n241 = Unbundle By Name(w433) -> ("ID"=w432:u32, "LEN"=w431:u8, "aDATA"=w430:u8[])
        n242 = case shown="15500008" w432 {
          tunnel: w430 -> [_ w437 _ w443 w447 w451 w454 w464 w475 w480 w488 w510]
          tunnel: w431 -> [_ _ _ _ _ _ _ _ _ _ _ _]
          tunnel: [_ _ _ _ _ _ _ _ _ _ _ TRUE] -> w429
          tunnel: w428 -> [w435 w436 w438 w439 w444 w448 w452 w455 w465 w476 w486 w501]
          tunnel: [w435 w436 w438 w439 w444 w448 w452 w455 w465 w476 w486 w501] -> w427
          frame 0, Default {
          }
          frame 357564416 {
            # "status"
            n243 = call "StatusReq.vi"("aDATA in"=w437) -> ()  [unwired: 1 in]
          }
          frame 357564417 {
            # "control"
          }
          frame 357564418 {
            # "ADC"
            n244 = call "ADCReq.vi"("aDATA"=w443, "Gain"="Gain", "Rsense"="Rsense") -> ("NumOut 1"=w440:dbl)  [unwired: 16 in]
            n245 = local write "ADC Units"(w440) -> ()
          }
          frame 357564420 {
            # "VinVout"
            n246 = call "Vin_Vout_Calc.vi"("aDATA"=w447) -> ("V in"=→"Vin [V]":dbl, "V Out"=→"Vout [V]":dbl)  [unwired: 1 out]
          }
          frame 357564423 {
            # "Version"
            n247 = call "Ver_PN.vi"("aDATA"=w451) -> ("Unit PN"=w450:string, "SW ver"=w449:string)
            n248 = local write "SW ver"(w449) -> ()
            n249 = local write "Unit PN"(w450) -> ()
          }
          frame 357564424 {
            n250 = call "Temp_Calc.vi"("aDATA"=w454) -> ("Temp CH 1-4"=w453:dbl)  [unwired: 1 in, 2 out]
            n251 = local write "Termistor"(w453) -> ()
          }
          frame 357564425 {
            n252 = local read "System Up Time"() -> (w463:u32)
            n253 = local read "Unit Add"() -> (w462:u32)
            n254 = local read "Op Amp Gain"() -> (w461:u32)
            n255 = local read "R Sense [Ohms]"() -> (w460:u32)
            n256 = call "SystemParams.vi"("aDATA"=w464, "R Sense [Ohms] in"=w460, "Op Amp Gain in"=w461, "Unit Add"=w462, "System Up Time In"=w463) -> ("Op Amp Gain out"=w456:u32, "R Sense [Ohms] out"=w457:u32, "Unit Add Out"=w458:u32, "System Up Time  Out"=w459:u32)  [unwired: 3 in]
            n257 = local write "System Up Time"(w459) -> ()
            n258 = local write "R Sense [Ohms]"(w456) -> ()
            n259 = local write "Unit Add"(w458) -> ()
            n260 = local write "Op Amp Gain"(w457) -> ()
          }
          frame 357564426 {
            n261 = local read "Channel On Delay [ms]"() -> (w472:u32)
            n262 = local read "Current Threshold [A]"() -> (w473:u32)
            n263 = local read "Number Of Retry"() -> (w467:u32)
            n264 = local read "Retry Delay"() -> (w468:u32)
            n265 = call "Single_ADC_Calc.vi"("aDATA"=w475, "Number Of Retry In"=w467, "Retry Delay In"=w468, "On Delay  In"=w472, "Current TH In"=w473) -> ("Retry Delay Out"=w470:u32, "Number Of Retry Out"=w469:u32, "On Delay Out"=w471:u32, "Current TH Out"=w474:u32, "CH R"=w466:u8)
            n266 = local write "Channel On Delay [ms]"(w471) -> ()
            n267 = local write "Current Threshold [A]"(w474) -> ()
            n268 = local write "Ch Received"(w466) -> ()
            n269 = local write "Number Of Retry"(w469) -> ()
            n270 = local write "Retry Delay"(w470) -> ()
          }
          frame 357564427 {
            n271 = Index Array(array=w480, index #1=0 ("index")) -> (element #1=w482:u8, element #2=w483:u8, element #3=w485:u8, element #4=w484:u8)  [unwired: 4 in, 1 out]
            n272 = Join Numbers(hi=w483, lo=w482) -> ((hi.lo)=w478:u16)
            n273 = Join Numbers(hi=w484, lo=w485) -> ((hi.lo)=w479:u16)
            n274 = Join Numbers(hi=w479, lo=w478) -> ((hi.lo)=→"Reset Counter":u32)
          }
          frame 357564428 {
            n275 = Index Array(array=w488, index #1=0 ("index")) -> (element #1=w492:u8, element #2=w493:u8, element #3=w495:u8, element #4=w494:u8)  [unwired: 4 in, 1 out]
            n276 = Join Numbers(hi=w493, lo=w492) -> ((hi.lo)=w489:u16)
            n277 = Join Numbers(hi=w494, lo=w495) -> ((hi.lo)=w490:u16)
            n278 = Join Numbers(hi=w490, lo=w489) -> ((hi.lo)=w487:u32)
            n279 = case shown="0" w487 {
              frame 0 {
                n280 = local write "Channel Protection"("ALL" ("Channel Protection")) -> ()
              }
              frame 1 {
                n281 = local write "Channel Protection"("ADC_OFF" ("Channel Protection")) -> ()
              }
              frame 2 {
                n282 = local write "Channel Protection"("FF_OFF" ("Channel Protection")) -> ()
              }
              frame 3 {
                n283 = local write "Channel Protection"("No Protection" ("Channel Protection")) -> ()
              }
              frame 4, Default {
                n284 = local write "Channel Protection"("In Valid Value" ("Channel Protection")) -> ()
              }
            }
          }
          frame 357564430 {
            n285 = local read "Event Logs"() -> (w508:string)
            n286 = local read "Rcv_Msg"() -> (w506:u8)
            n287 = call "Read_Logger.vi"("Input String"=w508, "Msg In"=w506, "aDATA"=w510) -> ("Output String"=w509:string, "End of Log"=w502:bool, "Msg out"=w505:u8, "Send_Msg"=w504:bool)
            n288 = Not(x=w502) -> (.not. x?=w503:bool)
            n289 = local write "Get_Log_Selector"(w503) -> ()
            n290 = local write "Send_Msg"(w504) -> ()
            n291 = local write "Rcv_Msg"(w505) -> ()
            n292 = local write "Event Logs"(w509) -> ()
          }
        }
      }
    }
    n293 = case shown="True" "cleanPl" {
      tunnel: [w422 cluster{"Time":timestamp, "Data":dbl}[] []] -> w414
      tunnel: w415 -> [w422 _]
      frame False {
      }
      frame True {
        n294 = local write "cleanPl"(FALSE ("clean  Ch 2")) -> ()
      }
    }
    "XY Graph" <- w414
  }
  n295 = while {
    tunnel: w9 -> [_]
    tunnel: ["RXFlagStop"] -> _
    tunnel: w1 -> [w513]
    shift-right: [w511] -> _
    shift-left: u32 0 -> [w512]
    stop <- "RXFlagStop" stop-if-true
    # "Receive Task"
    n296 = local read "CommIcon"() -> (w514:bool)
    n297 = case shown="False" w514 {
      tunnel: w513 -> [w519 _]
      tunnel: w512 -> [w518 w574]
      tunnel: [w517 w574] -> w511
      frame False {
        n298 = local read "CANType"() -> (w516:u16)
        n299 = case shown="3, 4" w516 {
          tunnel: w519 -> [w523 w553 w555 w563]
          tunnel: w518 -> [w521 w552 w556 w561]
          tunnel: [w520 w551 w557 w560] -> w517
          frame 1, Default {
            # "PCAN"
            n300 = call "PCAN_READ.vi"() -> ("error out"=w526:errorcluster, "TPCANMsg"=w524:T9, "error"=w525:T10)  [unwired: 2 in, 7 out]
            n301 = case shown="20" w525 {
              selector: w525 -> [w538 _ _]
              tunnel: w524 -> [_ w540 _]
              tunnel: w526 -> [w539 w546 w549]
              tunnel: [w537 w546 w549] -> w522
              tunnel: w523 -> [_ w545 _]
              tunnel: w521 -> [w529 w543 w547]
              tunnel: [w529 w542 w547] -> w520
              frame Default {
                n302 = call "PCAN_ERROR.vi"("error in (no error)"=w539, "Error Code"=w538) -> ("error out"=w537:errorcluster, "PCAN error"=w536:T11)  [unwired: 8 out]
                n303 = Wait (ms)(milliseconds to wait=u32 20) -> ()  [unwired: 1 out]
                n304 = Get Date/Time String() -> (date string=w534:string, time string=w533:string)  [unwired: 3 out]
                n305 = Unbundle By Name(w536) -> ("Message"=w532:string)
                n306 = call <vilib>:"Space Constant.vi"() -> ("String"=w531:string)
                n307 = Concatenate Strings(w534, w531, w533, w531, w532) -> (w527:string)
                "Error" <- w527
                n308 = local write "RX"(FALSE ("RX")) -> ()
                n309 = call "Str_Data.vi"("Err str"=w527, "string"="Err") -> ()  [unwired: 1 in, 1 out]
              }
              frame 0 {
                n310 = Unbundle By Name(w540) -> ()  [unwired: 4 out]
                n311 = Increment(x=w543) -> (x+1=w542:u32)
                n312 = local write "RX"(TRUE ("RX")) -> ()
                n313 = Enqueue Element(queue=w545, element=w540) -> ()  [unwired: 1 in, 4 out]
                n314 = call "Str_Data.vi"("Msg"=w540, "string"="RX") -> ()  [unwired: 1 in, 1 out]
                "MsgRX" <- w540
              }
              frame 32 {
                # "Wait if Buffer is empty"
                n315 = Wait (ms)(milliseconds to wait=u32 20) -> ()  [unwired: 1 out]
                n316 = local write "RX"(FALSE ("RX")) -> ()
              }
            }
            "error02" <- w522
          }
          frame 2 {
            # "CANalystII"
            n317 = control-ref of="Config_CANAT"() -> (w554:refnum<vi>)
            n318 = call "Reciev_CANATII.vi"("cnd_in"=w552, "queue out"=w553, "Config"=w554) -> ("cnt_out"=w551:u32)
          }
          frame 3, 4 {
            # "Eth Server/Client"
            n319 = control-ref of="conn ID"() -> (w558:refnum<vi>)
            n320 = call "ReceiveEth.vi"("Cnt in"=w556, "queue out"=w555, "reference"=w558) -> ("Cnt out"=w557:u32)
          }
          frame 0 {
            # "LAWICER"
            n321 = local read "VISA res_out"() -> (w566:refnum<visa-resource-name>)
            n322 = call "Read_CANUSB.vi"("VISA  in"=w566, "byte count"=u32 40) -> ("Status"=w559:bool, "TPCANMsg out"=w562:T9, "error out 5"=→"error out 5":errorcluster)  [unwired: 2 out]
            n323 = case shown="True" w559 {
              tunnel: w563 -> [_ w572]
              tunnel: w562 -> [_ w568]
              tunnel: w561 -> [w567 w571]
              tunnel: [w567 w570] -> w560
              frame False {
              }
              frame True {
                n324 = local write "MsgRX"(w568) -> ()
                n325 = Increment(x=w571) -> (x+1=w570:u32)
                n326 = local write "RX"(TRUE ("RX")) -> ()
                n327 = Enqueue Element(queue=w572, element=w568) -> ()  [unwired: 1 in, 4 out]
                n328 = call "Str_Data.vi"("Msg"=w568, "string"="RX") -> ()  [unwired: 1 in, 1 out]
              }
            }
          }
        }
      }
      frame True {
        n329 = Wait (ms)(milliseconds to wait=u32 10) -> ()  [unwired: 1 out]
      }
    }
    "RX Cnt" <- w511
  }
  n330 = flat-sequence {
    tunnel: w8 -> [w577]
    tunnel: w7 -> [w576]
    frame #0 {
      # "Exit"
      n331 = flat-sequence {
        tunnel: w577 -> [w582]
        tunnel: w576 -> [w579]
        frame #0 {
          n332 = local read "CANType"() -> (w578:u16)
          n333 = Release Queue(queue=w582) -> (error out=w581:errorcluster)  [unwired: 1 in, 3 out]
          n334 = Release Queue(queue=w579) -> (error out=w580:errorcluster)  [unwired: 1 in, 3 out]
          n335 = case shown="3, 4" w578 {
            frame 1, Default {
              # "PCAN"
              n336 = call "PCAN_CLOSE.vi"() -> ("error out"=→"error out 3":errorcluster)  [unwired: 1 in, 10 out]
            }
            frame 0 {
              # "LAWICER"
              n337 = flat-sequence {
                tunnel: [w586] -> w584
                tunnel: w584 -> [w590]
                frame #0 {
                  # "Close"
                  n338 = local read "VISA res_out"() -> (w586:refnum<visa-resource-name>)
                  n339 = call "SendData.vi"("String"="C", "byte count"=u32 20, "VISA resource name out 2"=w586) -> ("error out"=→"error out 7":errorcluster)  [unwired: 1 in, 3 out]
                }
                frame #1 {
                  n340 = VISA Close(VISA resource name=w590) -> (error out=→"erroro5 2":errorcluster)  [unwired: 1 in]
                }
              }
            }
            frame 2 {
              # "CANalystII"
              # "Close"
              n341 = local read "Config_CANAT"() -> (w592:T7)
              n342 = case shown="True" TRUE {
                tunnel: w592 -> [_ w593]
                frame False {
                }
                frame True {
                  n343 = Unbundle By Name(w593) -> ("DevType"=w595:T1, "DevIndex"=w594:u32)
                  n344 = call "VCI_CloseDevice.vi"("DevIndex"=w594, "DevType"=w595) -> ()  [unwired: 1 in, 9 out]
                }
              }
            }
            frame 3, 4 {
              w596 = FALSE ("status")
              n345 = local read "conn ID"() -> (w597:refnum<k5>)
              n346 = local write "status 2"(w596) -> ()
              n347 = local write "status"(w596) -> ()
              n348 = TCP Close Connection(connection ID=w597) -> ()  [unwired: 2 in, 2 out]
            }
          }
          n349 = call <vilib>:"Simple Error Handler.vi"("error in (no error)"=w581) -> ()  [unwired: 1 in, 8 out]
          n350 = call <vilib>:"Simple Error Handler.vi"("error in (no error)"=w580) -> ()  [unwired: 1 in, 8 out]
        }
        frame #1 {
          n351 = Wait (ms)(milliseconds to wait=u32 1000) -> ()  [unwired: 1 out]
        }
        frame #2 {
          n352 = Quit LabVIEW(quit? (T)=TRUE) -> ()
        }
      }
    }
  }
